vi "BRig_dataTrial_DAB_iSelect_HighProb.vi"() -> (2 "output_DAB_iSelect_HighProb":i32)   [LabVIEW 2014]
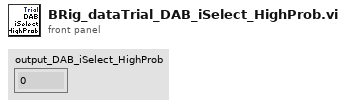
[diagram p1: front panel]
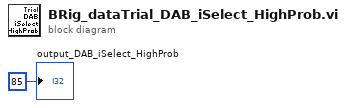
[diagram p0: block diagram]
diagram:
  "output_DAB_iSelect_HighProb" <- 85 ("output_iBlock")
